vi "set_iterations_per_pixel.vi"(8 "error in (no error)":errorcluster, 10 "iterations per pixel":i32, 11 "FPGAWrapperDL090211Galvo in":refnum<class "FPGAWrapperDL090211Galvo.lvclass">) -> (0 "error out":errorcluster, 3 "FPGAWrapperDL090211Galvo out":refnum<class "FPGAWrapperDL090211Galvo.lvclass">)   [LabVIEW 2010, in "FPGAWrapperDL090211Galvo.lvclass"]
uses:
  FPGAWrapperDL090211Galvo.lvclass
  FPGAWrapperDL090211Galvo.lvclass/FPGAWrapperDL090211Galvo.ctl
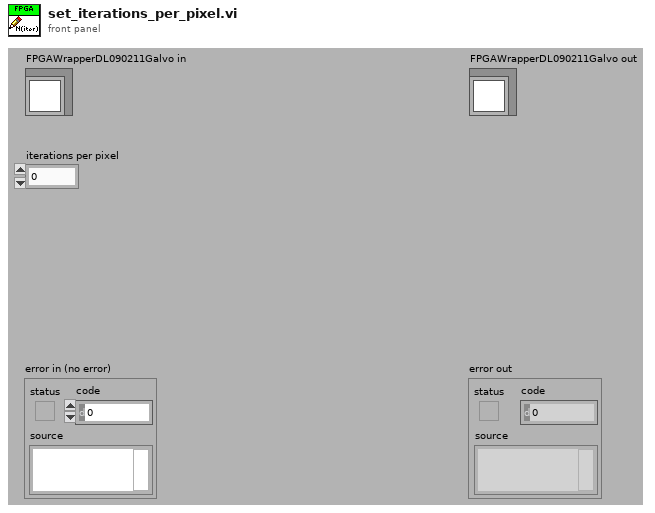
[diagram p1: front panel]
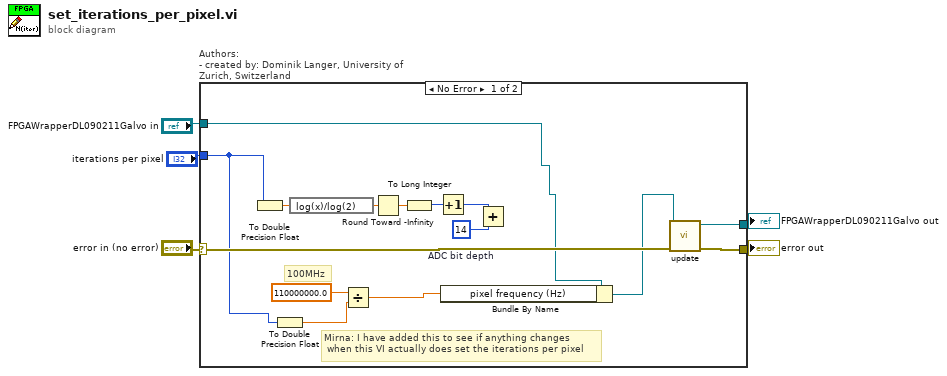
[diagram p0: block diagram]
diagram:
  n1 = case "Authors: \n- created by: Dominik Langer, University of Zurich, Switzerland" shown="No Error" "error in (no error)" {
    selector: "error in (no error)" -> [w14 w21]
    tunnel: "FPGAWrapperDL090211Galvo in" -> [w11 w22]
    tunnel: [w13 w22] -> w1
    tunnel: [w12 w21] -> w2
    tunnel: "iterations per pixel" -> [w7 _]
    frame No Error {
      w19 = 14  # ADC bit depth
      # "100MHz"
      # "Mirna: I have added this to see if anything changes\n when this VI actually does set the iterations per pixel"
      n2 = To Double Precision Float(number=w7) -> (double precision float=w16:dbl)
      n3 = To Double Precision Float(number=w7) -> (double precision float=w8:dbl)
      n4 = expression code="log(x)/log(2)"(w16) -> (w15:dbl)
      n5 = Divide(x=110000000.0, y=w8) -> (x/y=w9:dbl)
      n6 = Round Toward -Infinity(1:w15) -> (0:w20:dbl)
      n7 = To Long Integer(number=w20) -> (32bit integer=w18:i32)
      n8 = Increment(x=w18) -> (x+1=w17:i32)
      n9 = Bundle By Name(cluster=w11, "pixel frequency (Hz)"=w9) -> (w10:refnum<class "FPGAWrapperDL090211Galvo.lvclass">)
      n10 = Add(x=w17, y=w19) -> ()  [unwired: 1 out]
      n11 = call-dynamic "update.vi"("error in (no error)"=w14, "FPGAWrapperDL120115Galvo in"=w10) -> ("error out"=w12:errorcluster, "FPGAWrapperDL120115Galvo out"=w13:refnum<class "FPGAWrapperDL090211Galvo.lvclass">)  [unwired: 8 in]
    }
    frame Error {
    }
  }
  "error out" <- w2
  "FPGAWrapperDL090211Galvo out" <- w1
